vi "AOoutput.vi"(8 "error in (no error)":errorcluster caption="错误输入（无错误）", 10 "波形参数":cluster{"波形类型":u16, "幅值":dbl, "频率":dbl}[](array[cluster])=[{"波形类型"=0, "幅值"=1.0, "频率"=10.0}] {"频率" format="%0.2p"; "幅值" format="%0.2p"; "波形类型" items=["正弦波", "三角波", "方波", "锯齿波"]}, 11 "Hardware Resources in":T1 caption="硬件资源输入") -> (0 "error out":errorcluster caption="错误输出", 2 "波形图":waveform(dbl)[](graph)=[{"t0"=timestamp(0 s since 1904-01-01), "dt"=0.001, "Y"=[]}], 3 "Hardware Resources out":T1 caption="硬件资源输出")   [LabVIEW 2014]
uses:
  Hardware Configures.ctl
  <vilib>/DAQmx/write.llb/DAQmx Write (Analog 1D Wfm NChan NSamp).vi
  <vilib>/DAQmx/miscellaneous.llb/DAQmx Fill In Error Info.vi
  <vilib>/measure/NI_MABase.lvlib
  HardWareConfig.lvlib
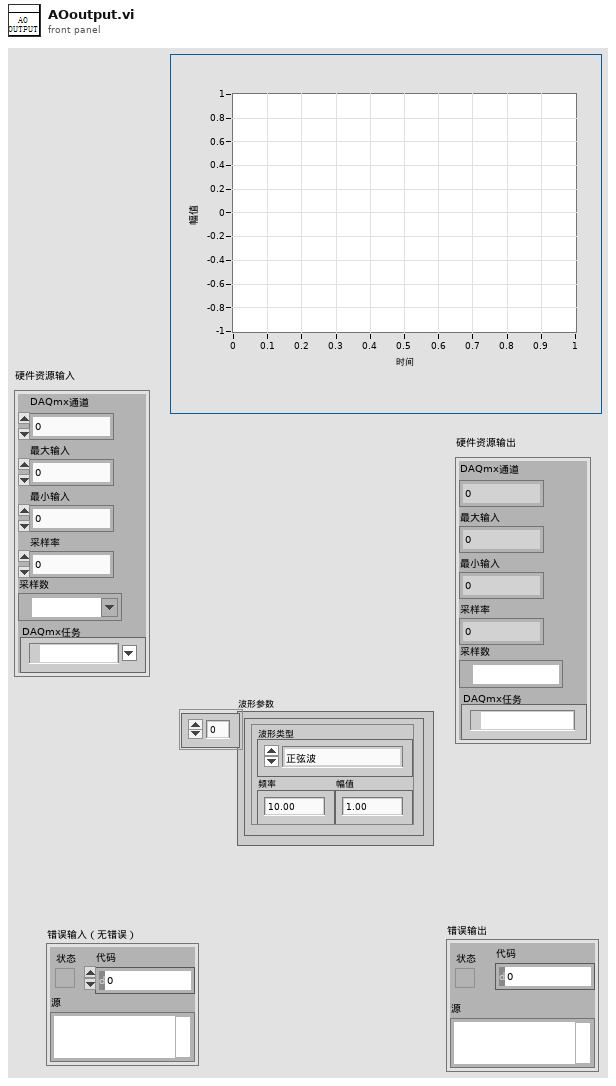
[diagram p1: front panel]
types:
  T1 = typedef "HardWareConfig.lvlib/Hardware Configures.ctl" = cluster{"Max Input":dbl, "Min Input":dbl, "Sample Rate":dbl, "Sample Num":dbl, "DAQmx Task":refnum<k21>, "物理通道":tag}
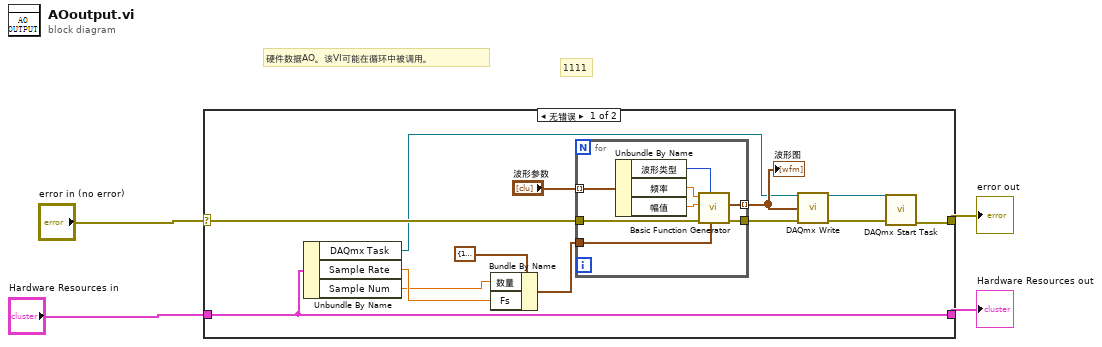
[diagram p0: block diagram]
diagram:
  # "1111"
  # "硬件数据AO。该VI可能在循环中被调用。"
  n1 = case shown="无错误" "error in (no error)" {
    selector: "error in (no error)" -> [w11 w26]
    tunnel: [w5 w26] -> w3
    tunnel: "Hardware Resources in" -> [w17 w27]
    tunnel: [w17 w27] -> w1
    frame No Error {
      n2 = Unbundle By Name(w17) -> ("DAQmx Task"=w10:refnum<k21>, "Sample Rate"=w9:dbl, "Sample Num"=w8:dbl)
      n3 = Bundle By Name(cluster=cluster{"Fs":dbl, "数量":dbl} {"Fs"=1000.0, "数量"=1000.0} ("采样信息"), "数量"=w8, "Fs"=w9) -> (w15:cluster{"Fs":dbl, "数量":dbl})
      n4 = for {
        tunnel: w15 -> [w25]
        tunnel: [w24] -> w14
        tunnel: "波形参数" -> [w23] mode=indexing
        tunnel: [w19] -> w12 mode=indexing
        tunnel: w11 -> [w18]
        n5 = Unbundle By Name(w23) -> ("波形类型"=w22:u16, "频率"=w21:dbl, "幅值"=w20:dbl)
        n6 = call <vilib>:"Basic Function Generator.vi"("sampling info"=w25, "signal type"=w22, "error in (no error)"=w18, "amplitude"=w20, "frequency"=w21) -> ("error out"=w24:errorcluster, "signal out"=w19:waveform(dbl))  [unwired: 4 in, 1 out]
      }
      "波形图" <- w12
      n7 = call-poly <vilib>:"DAQmx Write.vi"("task/channels in"=w10, "data"=w12, "error in"=w14) -> ("task out"=w7:refnum<k21>, "error out"=w6:errorcluster)  [unwired: 10 in, 1 out]
      n8 = call <vilib>:"DAQmx Start Task.vi"("task/channels in"=w7, "error in"=w6) -> ("error out"=w5:errorcluster)  [unwired: 12 in, 1 out]
    }
    frame Error {
    }
  }
  "Hardware Resources out" <- w1
  "error out" <- w3
